vi "set_env_variable.vi"(6 "Value":string, 7 "Environment Variable Name":string="labview_llm_openai_key") -> (0 "error out":errorcluster)   [LabVIEW 2020]
uses:
  <vilib>/Utility/config.llb/Write Key (String).vi
  <vilib>/Utility/config.llb/NI_LVConfig.lvlib
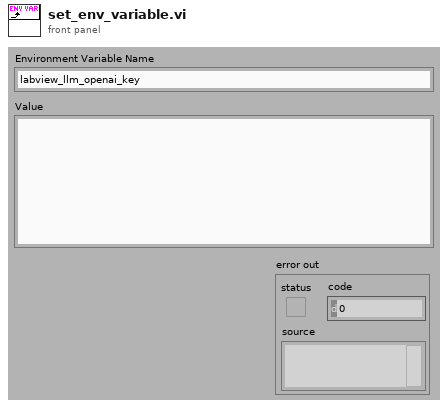
[diagram p1: front panel]
types:
  T1 = typedef "NI_LVConfig.lvlib/Config Data RefNum.ctl" = refnum<k1>
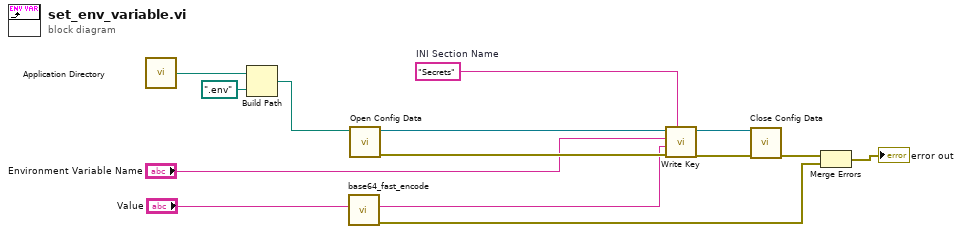
[diagram p0: block diagram]
diagram:
  w13 = "Secrets"  # INI Section Name
  n1 = call <vilib>:"Application Directory.vi"() -> ("Application Directory"=w11:path)
  n2 = Build Path(base path=w11, name or relative path=path ".env") -> (appended path=w9:path)
  n3 = call "base64_fast_encode.vi"("string in (not encoded)"="Value") -> ("error out"=w1:errorcluster, "string out (base64-encoded)"=w3:string)  [unwired: 9 in]
  n4 = call <vilib>:"Open Config Data.vi"("configuration file path"=w9) -> ("error out"=w14:errorcluster, "refnum"=w12:T1)  [unwired: 8 in, 1 out]
  n5 = call-poly <vilib>:"Write Key.vi"("section"=w13, "error in (no error)"=w14, "value"=w3, "key"="Environment Variable Name", "refnum"=w12) -> ("error out"=w6:errorcluster, "refnum out"=w7:T1)  [unwired: 4 in, 1 out]
  n6 = call <vilib>:"Close Config Data.vi"("error in (no error)"=w6, "refnum"=w7) -> ("error out"=w5:errorcluster)  [unwired: 8 in, 1 out]
  n7 = Merge Errors(w5, w1) -> (→"error out":errorcluster)
